vi "Process_POST.vi"(11 "LabVIEW Web Service Request":refnum<class "Web Request.lvclass">) -> ()   [LabVIEW 2013]
uses:
  <vilib>/wsapi/Web Request.lvclass
  ScoreEntry.ctl
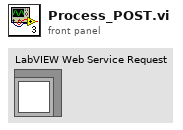
[diagram p1: front panel]
types:
  T1 = typedef "ScoreEntry.ctl" = cluster{"Elements":cluster{"Name":string, "Value":string}[], "Score":dbl}
  T2 = typedef "Team Data.ctl" = cluster{"Both":string, "Name":string, "GUID":u16, "Number":u16}
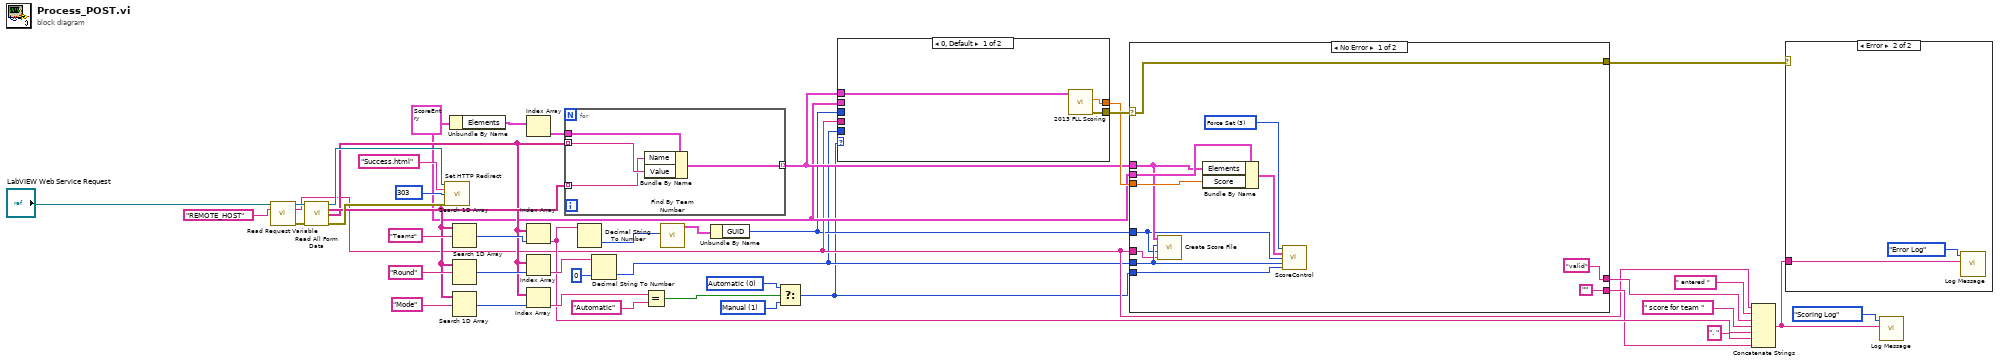
[diagram p0: block diagram]
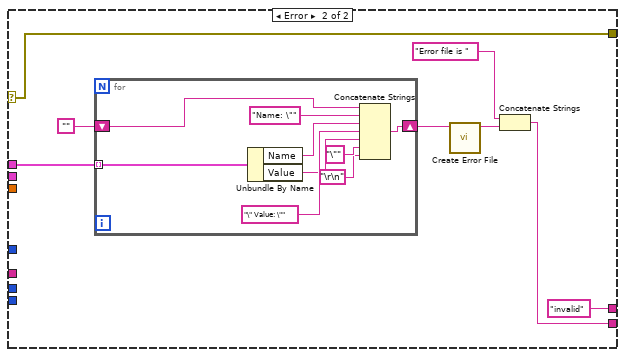
[diagram p2: hidden frame]
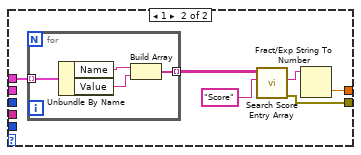
[diagram p4: hidden frame]
diagram:
  w5 = T1 {"Elements"=[{"Name"="CO2 Balls Touching/Within Reservoir Model", "Value"="-1"}, {"Name"="Money Ball Touching/Within Reservoir Model", "Value"="-1"}, {"Name"="3+ Red/White Citizens in Pink Grid Area", "Value"="-1"}, {"Name"="# Upright Levee Blocks touching ONLY GREEN shores", "Value"="-1"}, {"Name"="# Upright Levee Blocks Touching any RED shore", "Value"="-1"}, {"Name"="Levee Test was Performed", "Value"="-1"}, {"Name"="Levee Test Wheel Blocked by NonLevee", "Value"="-1"}, {"Name"="Flood Barrier in Up Position", "Value"="-1"}, {"Name"="Both Yellow Arrows Aligned", "Value"="-1"}, {"Name"="Team Robot Touching Only Yellow Grid Area", "Value"="-1"}, {"Name"="Both Insulation Touching Green Grid Area", "Value"="-1"}, {"Name"="Bicycle Touching Green Grid Area", "Value"="-1"}, {"Name"="Computer Touching Green Grid Area", "Value"="-1"}, {"Name"="House in Up Position", "Value"="-1"}, {"Name"="House Window Showing Black", "Value"="-1"}, {"Name"="House Window All The Way Open", "Value"="-1"}, {"Name"="3+ Black/White Scientists Touching Research Area", "Value"="-1"}, {"Name"="Money Ball Touching/Within Research Area Model", "Value"="-1"}, {"Name"="Polar Bear Touching/Within Research Area Model", "Value"="-1"}, {"Name"="Polar Bear Orientation (Sleeping/Upright)", "Value"="-1"}, {"Name"="Ice Core Pulled From Its Hole", "Value"="-1"}, {"Name"="Ice Buoy Upright and Within/Touching Research Area Model", "Value"="-1"}, {"Name"="Drilling Machine Touching/Within Research Area Model", "Value"="-1"}, {"Name"="Drill Assembly Completely Vertical", "Value"="-1"}, {"Name"="Team Robot Touching/Within Research Area Model", "Value"="-1"}, {"Name"="3+ Blue/Gray Leaders Touching Green Mountain/City Area", "Value"="-1"}, {"Name"="Ice Core in Base Area", "Value"="-1"}, {"Name"="Snowmobile Touching/Within Research Area Model", "Value"="-1"}], "Score"=0.0} ("Full Score Entry")
  w26 = u16 1 items=["Automatic", "Manual"] ("Score Mode Selector")
  w27 = u16 0 items=["Automatic", "Manual"] ("Score Mode Selector")
  w43 = 303 items=["100"=100, "101"=101, "200"=200, "201"=201, "202"=202, "203"=203, "204"=204, "205"=205, "206"=206, "300"=300, "301"=301, "302"=302, "303"=303, "304"=304, "305"=305, "306"=306, "307"=307, "400"=400, "401"=401, "402"=402, "403"=403, "404"=404, "405"=405, "406"=406, "407"=407, "408"=408, "409"=409, "410"=410, "411"=411, "412"=412, "413"=413, "414"=414, "415"=415, "416"=416, "417"=417, "500"=500, "501"=501, "502"=502, "503"=503, "504"=504, "505"=505] ("response code (307)")
  n1 = call <vilib>:"Read Request Variable.vi"("LabVIEW Web Service Request"="LabVIEW Web Service Request", "variable name"="REMOTE_HOST") -> ("LabVIEW Web Service Request out"=w20:refnum<class "Web Request.lvclass">, "value"=w4:string, "error out"=w18:errorcluster)  [unwired: 11 in]
  n2 = call <vilib>:"Read All Form Data.vi"("LabVIEW Web Service Request"=w20, "error in (no error)"=w18) -> ("LabVIEW Web Service Request out"=w44:refnum<class "Web Request.lvclass">, "Key"=w32:string[], "Value"=w31:string[], "error out"=w42:errorcluster)  [unwired: 9 in, 1 out]
  n3 = call <vilib>:"Set HTTP Redirect.vi"("LabVIEW Web Service Request"=w44, "redirect URL"="Success.html", "response code (307)"=w43, "error in (no error)"=w42) -> ()  [unwired: 10 in, 2 out]
  n4 = Unbundle By Name(w5) -> ("Elements"=w25:cluster{"Name":string, "Value":string}[])
  n5 = Search 1D Array(1D array=w32, element="Teams") -> (index of element=w38:i32)  [unwired: 1 in]
  n6 = Search 1D Array(1D array=w32, element="Round") -> (index of element=w40:i32)  [unwired: 1 in]
  n7 = Search 1D Array(1D array=w32, element="Mode") -> (index of element=w33:i32)  [unwired: 1 in]
  n8 = Index Array(array=w25) -> (element=w24:cluster{"Name":string, "Value":string})  [unwired: 1 in]
  n9 = Index Array(array=w31, index=w38) -> (element=w12:string)
  n10 = Index Array(array=w31, index=w40) -> (element=w39:string)
  n11 = Index Array(array=w31, index=w33) -> (element=w30:string)
  n12 = for {
    tunnel: w32 -> [w46] mode=indexing
    tunnel: w31 -> [w48] mode=indexing
    tunnel: [w47] -> w6 mode=indexing
    tunnel: w24 -> [w45]
    n13 = Bundle By Name(cluster=w45, "Name"=w46, "Value"=w48) -> (w47:cluster{"Name":string, "Value":string})
  }
  n14 = Decimal String To Number(string=w12) -> (number=w36:i32)  [unwired: 2 in, 1 out]
  n15 = Decimal String To Number(string=w39, default (0L)=u16 0) -> (number=w2:u16)  [unwired: 1 in, 1 out]
  n16 = Equal?(x=w30, y="Automatic") -> (x = y?=w28:bool)
  n17 = call "Find By Team Number.vi"("Team Number"=w36) -> ("Team Data"=w22:T2)  [unwired: 9 in, 1 out]
  n18 = Unbundle By Name(w22) -> ("GUID"=w3:u16)
  n19 = Select(t=w27, s=w28, f=w26) -> (s? t:f=w1:u16)
  n20 = case shown="0, Default" w1 {
    tunnel: w2 -> [_ _]
    tunnel: w5 -> [_ _]
    tunnel: w3 -> [_ _]
    tunnel: w6 -> [w51 w54]
    tunnel: w4 -> [_ _]
    tunnel: [w50 w53] -> w9
    tunnel: [w49 w52] -> w8
    frame 0, Default {
      n21 = call "2013 FLL Scoring.vi"("Array"=w51) -> ("error out"=w50:errorcluster, "Total Score"=w49:dbl)  [unwired: 9 in]
    }
    frame 1 {
      n22 = for {
        tunnel: w54 -> [w61] mode=indexing
        tunnel: [w58] -> w57 mode=indexing
        n23 = Unbundle By Name(w61) -> ("Name"=w60:string, "Value"=w59:string)
        n24 = Build Array(w60, w59) -> (w58:string[])
      }
      n25 = call "Search Score Entry Array.vi"("Item Name"="Score", "Array"=w57) -> ("error out"=w53:errorcluster, "Value"=w55:string)  [unwired: 6 in, 2 out]
      n26 = Fract/Exp String To Number(string=w55) -> (number=w52:dbl)  [unwired: 3 in, 1 out]
    }
  }
  n27 = case shown="No Error" w9 {
    selector: w9 -> [w62 w74]
    tunnel: w2 -> [w65 _]
    tunnel: w1 -> [w72 _]
    tunnel: w5 -> [w71 _]
    tunnel: w3 -> [w64 _]
    tunnel: w6 -> [w66 w78]
    tunnel: ["valid" ("string") "invalid" ("string")] -> w10
    tunnel: ["" w79] -> w11
    tunnel: w8 -> [w67 _]
    tunnel: w4 -> [w63 _]
    tunnel: [w62 w74] -> w7
    frame No Error {
      w73 = u16 3 items=["Get All", "Set", "Reset All", "Force Set"] ("Get/Set Mode Selector")
      n28 = call "Create Score File.vi"("Submitter"=w63, "GUID"=w64, "Round"=w65, "Scoring Data"=w66) -> ()  [unwired: 8 in]
      n29 = Bundle By Name(cluster=w71, "Elements"=w66, "Score"=w67) -> (w70:T1)
      n30 = call "ScoreControl.vi"("Get/Set Mode Selector"=w73, "Full Score Entry"=w70, "GUID"=w64, "Round Number"=w65, "Score Mode Selector"=w72) -> ()  [unwired: 9 in, 2 out]
    }
    frame Error {
      n31 = for {
        tunnel: w78 -> [w90] mode=indexing
        shift-right: [w82] -> w76
        shift-left: "" -> [w83]
        n32 = Unbundle By Name(w90) -> ("Name"=w88:string, "Value"=w86:string)
        n33 = Concatenate Strings(w83, "Name: \"" ("string"), w88, "\" Value: \"" ("string"), w86, "\"" ("string"), "\r\n") -> (w82:string)
      }
      n34 = call "Create Error File.vi"("File Contents"=w76) -> ("Filename"=w75:string)  [unwired: 10 in]
      n35 = Concatenate Strings("Error file is " ("string"), w75) -> (w79:string)
    }
  }
  n36 = Concatenate Strings(w4, " entered " ("string"), w10, " score for team " ("string"), w12, ". " ("string"), w11) -> (w13:string)
  n37 = case shown="Error" w7 {
    tunnel: w13 -> [_ w91]
    frame No Error {
    }
    frame Error {
      n38 = call "Log Message.vi"("Message"=w91, "Log"=enum16{"Error Log", "Timer Log", "Scoring Log"}."Error Log") -> ()  [unwired: 10 in]
    }
  }
  n39 = call "Log Message.vi"("Message"=w13, "Log"=enum16{"Error Log", "Timer Log", "Scoring Log"}."Scoring Log") -> ()  [unwired: 10 in]
